vi "Teleop.vi"() -> ()   [LabVIEW 2018]
doc: "This VI is called for each TeleOp packet received from the DS where the robot is not disabled. It is often used to read from the joysticks and update I/O or to update setpoints for timed control loops. It should complete and return within 20 milliseconds or it may miss DS packets."
uses:
  <vilib>/Rock Robotics/Network Tables/NT Read Numeric Array.vi
  <vilib>/Rock Robotics/WPI/Utilities/WPI_GetSetVariantRefNum.vi
  <vilib>/Rock Robotics/Network Tables/NT Write Numeric Array.vi
panel:
  out "Num Bytes Written":u32
  in  "Send LED Byte":bool
  in  "LED Byte":string
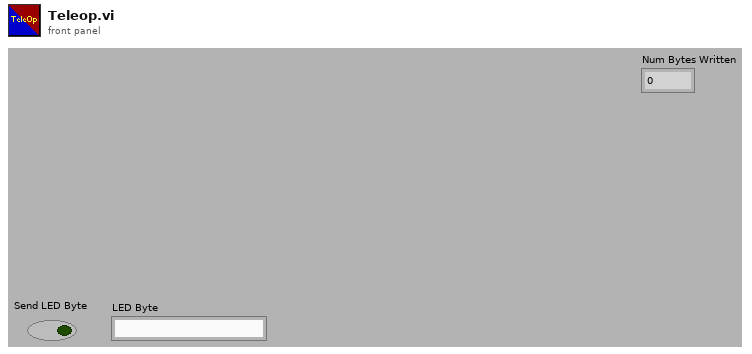
[diagram p1: front panel]
types:
  T1 = typedef "WPI_JoystickDevRef.ctl" = cluster{"Device":T2}
  T2 = typedef "WPI_JoystickDeviceEnum.ctl" = enum16{"USB 0", "USB 1", "USB 2", "USB 3", "USB 4", "USB 5"}
  T3 = typedef "WPI_MotorControlDeviceRef.ctl" = cluster{"DeviceStatus":errorcluster, "Type":T4, "PWM":cluster{"PWM Channel":T5, "DeadBand":T6}, "CAN":cluster{"Device Number":u8, "SetOutput VI Ref":variant, "GetOutput VI Ref":variant, "Enable VI Ref":variant, "Disable VI Ref":variant, "Data":variant}, "Invert":bool, "DIO PWM":cluster{"PWM \"Enable\" Channel":T5, "DIOChannel":T7, "PWM Rate":dbl}}
  T4 = typedef "WPI_MotorControlType.ctl" = enum16{"PWM", "CAN", "DIO PWM"}
  T5 = typedef "FPGA_DIOPWMChannel.ctl" = enum8{"PWM 0", "PWM 1", "PWM 2", "PWM 3", "PWM 4", "PWM 5", "PWM 6", "PWM 7", "PWM 8", "PWM 9", "PWM MXP 0", "PWM MXP 1", "PWM MXP 2", "PWM MXP 3", "PWM MXP 4", "PWM MXP 5", "PWM MXP 6", "PWM MXP 7", "PWM MXP 8", "PWM MXP 9", "Invalid"}
  T6 = typedef "WPI_PWMDeadband.ctl" = cluster{"Name":string, "maxPositivePwm":i32, "minPositivePwm":i32, "centerPwm":i32, "maxNegativePwm":i32, "minNegativePwm":i32, "angularRange":u16}
  T7 = typedef "FPGA_DIOChannel.ctl" = enum8{"DIO 0", "DIO 1", "DIO 2", "DIO 3", "DIO 4", "DIO 5", "DIO 6", "DIO 7", "DIO 8", "DIO 9", "DIO MXP 0", "DIO MXP 1", "DIO MXP 2", "DIO MXP 3", "DIO MXP 4", "DIO MXP 5", "DIO MXP 6", "DIO MXP 7", "DIO MXP 8", "DIO MXP 9", "DIO MXP 10", "DIO MXP 11", "DIO MXP 12", "DIO MXP 13", "DIO MXP 14", "DIO MXP 15", "SPI Port CS1", "SPI Port CS2", "SPI Port CS3", "SPI Port MISO", "SPI Port MOSI", "Invalid"}
  T8 = typedef "WPI_SerialPortRef.ctl" = cluster{"DevStatus":errorcluster, "Serial Port Name":refnum<visa-resource-name>}
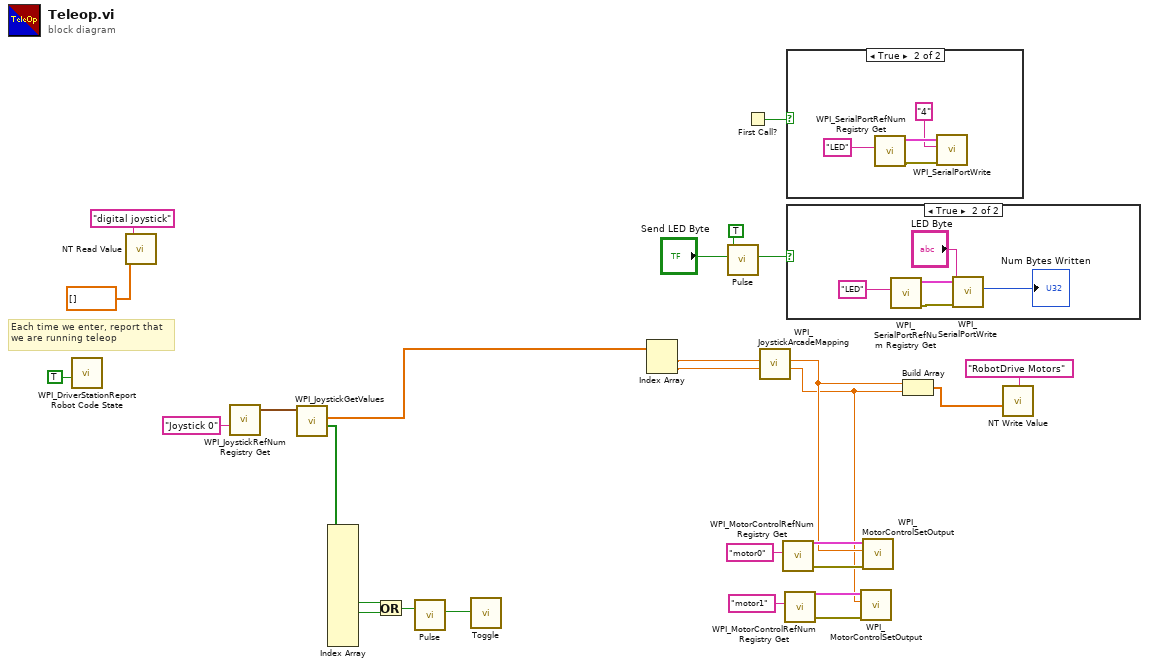
[diagram p0: block diagram]
diagram:
  # "Each time we enter, report that\nwe are running teleop"
  n1 = call <vilib>:"WPI_DriverStationReport Robot Code State.vi"("TeleOp"=TRUE ("Autonomous")) -> ()  [unwired: 10 in, 1 out]
  n2 = call-poly <vilib>:"NT Read Value.vi"("Default Value"=dbl[] [], "Name"="digital joystick") -> ()  [unwired: 8 in, 2 out]
  n3 = call <vilib>:"WPI_JoystickRefNum Registry Get.vi"("refnum name"="Joystick 0") -> ("JoystickDevRef"=w19:T1)  [unwired: 9 in, 1 out]
  n4 = call <vilib>:"WPI_JoystickGetValues.vi"("JoystickDevRef"=w19) -> ("Buttons"=w17:bool[], "Axes"=w18:dbl[])  [unwired: 6 in, 3 out]
  n5 = Index Array(array=w17) -> (element #8=w16:bool, element #9=w15:bool)  [unwired: 13 in, 11 out]
  n6 = Or(x=w16, y=w15) -> (x .or. y?=w14:bool)
  n7 = call "Pulse.vi"("Input"=w14) -> ("Output"=w13:bool)  [unwired: 10 in]
  n8 = call "Toggle.vi"("Input"=w13) -> ()  [unwired: 10 in, 1 out]
  n9 = Index Array(array=w18) -> (element #1=w24:dbl, element #2=w23:dbl)  [unwired: 2 in]
  n10 = call "Pulse.vi"("Input"="Send LED Byte", "Rising Edge?"=TRUE) -> ("Output"=w12:bool)  [unwired: 9 in]
  n11 = First Call?() -> (First Call?: T/F=w11:bool)
  n12 = call <vilib>:"WPI_JoystickArcadeMapping.vi"("Y axis value"=w23, "X axis value"=w24) -> ("Right Motor Value"=w1:dbl, "Left Motor Value"=w4:dbl)  [unwired: 8 in]
  n13 = call <vilib>:"WPI_MotorControlRefNum Registry Get.vi"("refnum name"="motor0") -> ("error out"=w5:errorcluster, "MotorControlDevRef"=w6:T3)  [unwired: 9 in]
  n14 = call <vilib>:"WPI_MotorControlRefNum Registry Get.vi"("refnum name"="motor1") -> ("error out"=w2:errorcluster, "MotorControlDevRef"=w3:T3)  [unwired: 9 in]
  n15 = case shown="True" w11 {
    frame False {
    }
    frame True {
      n16 = call <vilib>:"WPI_SerialPortRefNum Registry Get.vi"("refnum name"="LED") -> ("error out"=w28:errorcluster, "SerialPortRef"=w30:T8)  [unwired: 9 in]
      n17 = call <vilib>:"WPI_SerialPortWrite.vi"("error in (no error)"=w28, "Buffer"="4", "SerialPortRef"=w30) -> ()  [unwired: 6 in, 3 out]
    }
  }
  n18 = case shown="True" w12 {
    frame False {
    }
    frame True {
      n19 = call <vilib>:"WPI_SerialPortRefNum Registry Get.vi"("refnum name"="LED") -> ("error out"=w34:errorcluster, "SerialPortRef"=w35:T8)  [unwired: 9 in]
      n20 = call <vilib>:"WPI_SerialPortWrite.vi"("error in (no error)"=w34, "Buffer"="LED Byte", "SerialPortRef"=w35) -> ("Num Bytes Written"=→"Num Bytes Written":u32)  [unwired: 6 in, 2 out]
    }
  }
  n21 = call <vilib>:"WPI_MotorControlSetOutput.vi"("error in (no error)"=w2, "Output"=w1, "MotorControlDevRef"=w3) -> ()  [unwired: 6 in, 3 out]
  n22 = call <vilib>:"WPI_MotorControlSetOutput.vi"("error in (no error)"=w5, "Output"=w4, "MotorControlDevRef"=w6) -> ()  [unwired: 6 in, 3 out]
  n23 = Build Array(w4, w1) -> (w22:dbl[])
  n24 = call-poly <vilib>:"NT Write Value.vi"("Numeric Array"=w22, "Name"="RobotDrive Motors") -> ()  [unwired: 9 in, 1 out]
